vi "deeplabv3_opencv.vi"() -> ()   [LabVIEW 2018]
uses:
  <vilib>/addons/VIRobotics/opencv_yiku/ctls/ColorConversionCodes.ctl
  <vilib>/addons/VIRobotics/opencv_yiku/Mat/Mat_32F/Mat_32F.lvclass
  C:/Program Files/National Instruments/LabVIEW 2018_64bit/vi.lib/addons/VIRobotics/opencv_yiku/Mat/Mat/Mat.lvclass
  <vilib>/addons/VIRobotics/opencv_yiku/Mat/Mat_8U/Mat_8U.lvclass
  <vilib>/addons/VIRobotics/opencv_yiku/Mat/Mat/Mat_length.vi
  <vilib>/addons/VIRobotics/opencv_yiku/Mat/Mat/Mat_release.vi
  <vilib>/addons/VIRobotics/opencv_yiku/dnn/Net/Net.lvclass
  <vilib>/addons/VIRobotics/opencv_yiku/opencv_yiku.lvlib
  <vilib>/addons/VIRobotics/opencv_yiku/Mat/Mat/Mat.lvclass
panel:
  out "mask":picture
  out "原始图像":picture
  out "合成的图像":picture
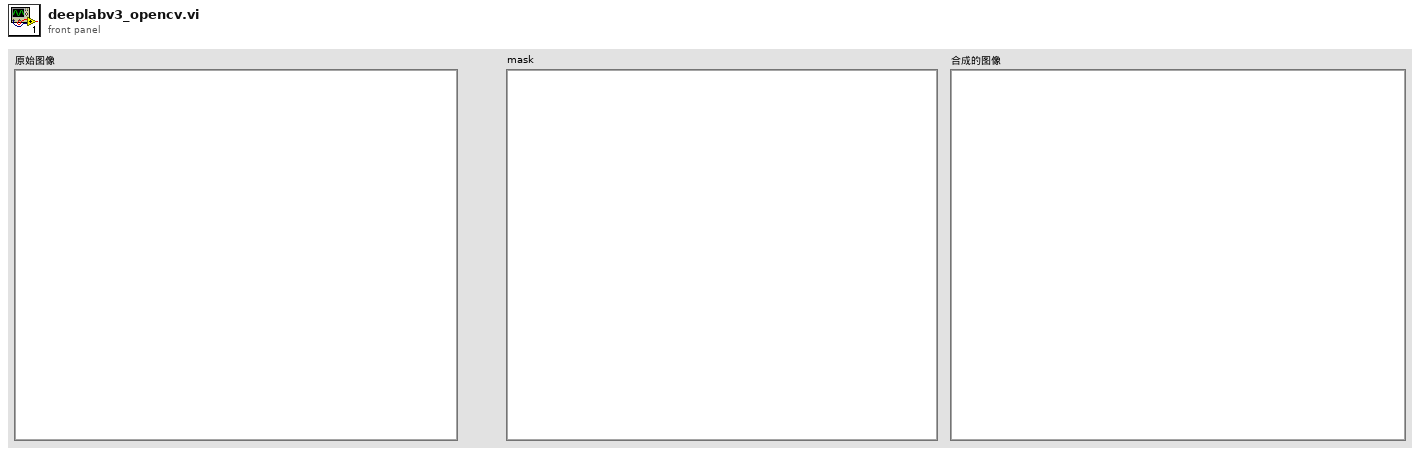
[diagram p1: front panel]
types:
  T1 = typedef "opencv_yiku.lvlib/ColorConversionCodes.ctl" = enum32{"COLOR_BGR2BGRA", "COLOR_BGRA2BGR", "COLOR_BGR2RGBA", "COLOR_RGBA2BGR", "COLOR_BGR2RGB", "COLOR_BGRA2RGBA", "COLOR_BGR2GRAY", "COLOR_RGB2GRAY", "COLOR_GRAY2BGR", "COLOR_GRAY2BGRA", "COLOR_BGRA2GRAY", "COLOR_RGBA2GRAY", "COLOR_BGR2BGR565", "COLOR_RGB2BGR565", "COLOR_BGR5652BGR", "COLOR_BGR5652RGB", "COLOR_BGRA2BGR565", "COLOR_RGBA2BGR565", "COLOR_BGR5652BGRA", "COLOR_BGR5652RGBA", "COLOR_GRAY2BGR565", "COLOR_BGR5652GRAY", "COLOR_BGR2BGR555", "COLOR_RGB2BGR555", "COLOR_BGR5552BGR", "COLOR_BGR5552RGB", "COLOR_BGRA2BGR555", "COLOR_RGBA2BGR555", "COLOR_BGR5552BGRA", "COLOR_BGR5552RGBA", "COLOR_GRAY2BGR555", "COLOR_BGR5552GRAY", "COLOR_BGR2XYZ", "COLOR_RGB2XYZ", "COLOR_XYZ2BGR", "COLOR_XYZ2RGB", "COLOR_BGR2YCrCb", "COLOR_RGB2YCrCb", "COLOR_YCrCb2BGR", "COLOR_YCrCb2RGB", "COLOR_BGR2HSV", "COLOR_RGB2HSV", "42", "43", "COLOR_BGR2Lab", "COLOR_RGB2Lab"}
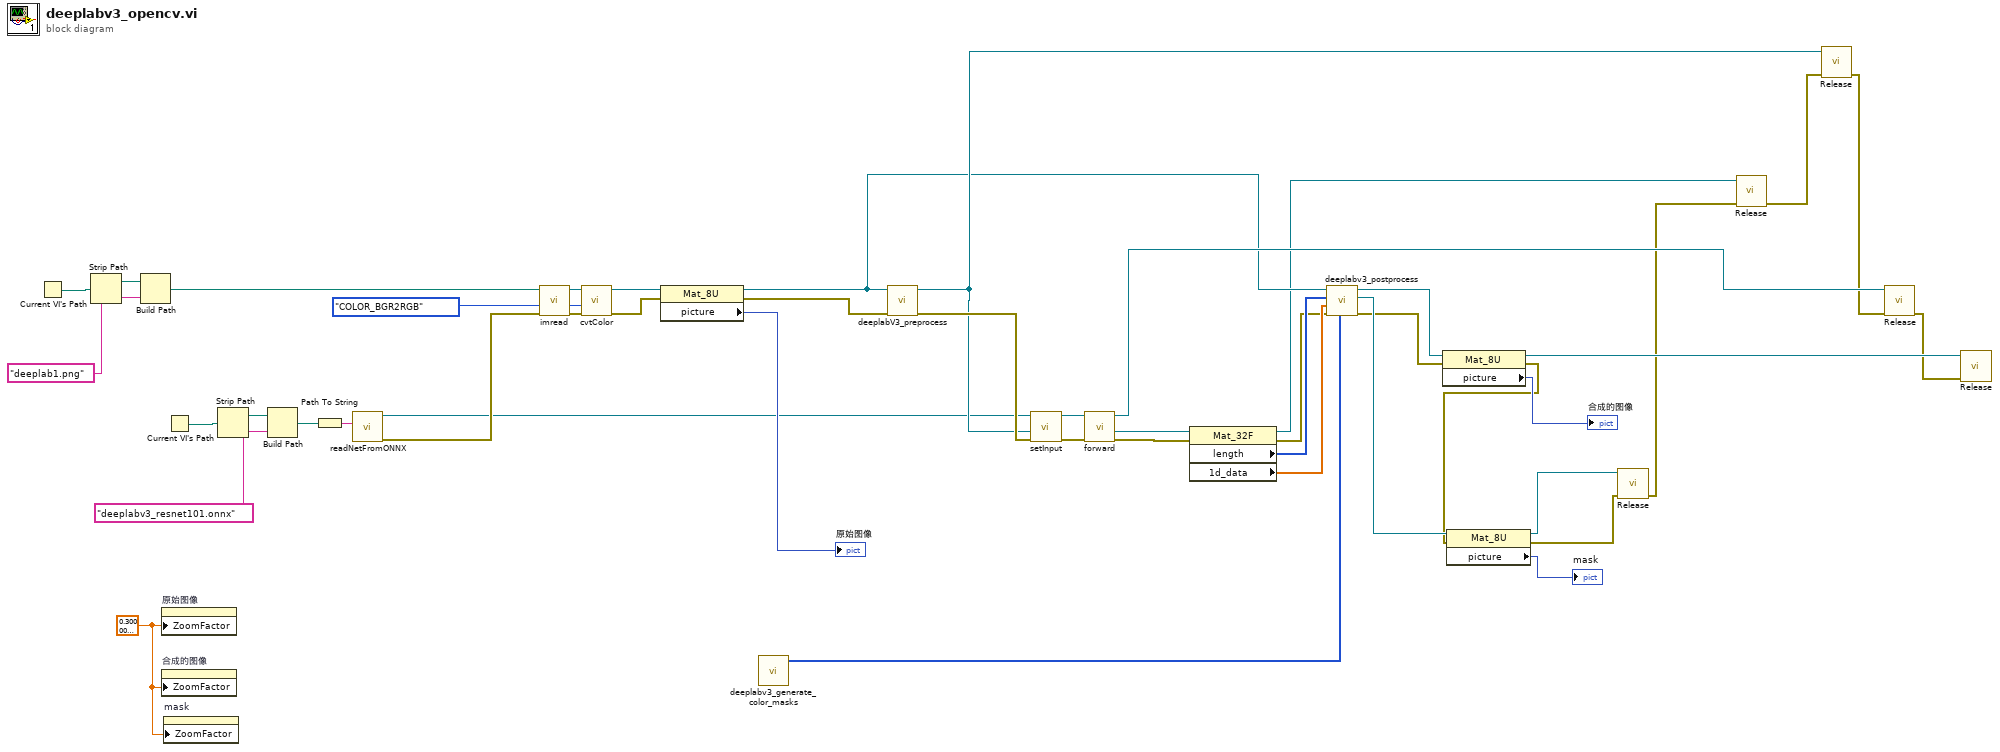
[diagram p0: block diagram]
diagram:
  w14 = sgl 0.3 ("Zoom Factor")
  n1 = Current VI's Path() -> (path=w41:path)
  n2 = Strip Path(path=w41) -> (stripped path=w42:path)  [unwired: 1 out]
  n3 = Build Path(base path=w42, name or relative path="deeplab1.png") -> (appended path=w39:path)
  n4 = property on="原始图像" class="Pict"("ZoomFactor"=w14) -> ()  [unwired: 2 in, 2 out]
  n5 = property on="合成的图像" class="Pict"("ZoomFactor"=w14) -> ()  [unwired: 2 in, 2 out]
  n6 = property on="mask" class="Pict"("ZoomFactor"=w14) -> ()  [unwired: 2 in, 2 out]
  n7 = Current VI's Path() -> (path=w37:path)
  n8 = Strip Path(path=w37) -> (stripped path=w38:path)  [unwired: 1 out]
  n9 = Build Path(base path=w38, name or relative path="deeplabv3_resnet101.onnx") -> (appended path=w35:path)
  n10 = Path To String(path=w35) -> (string=w45:string)
  n11 = call <vilib>:"readNetFromONNX.vi"("model"=w45) -> ("error out"=w43:errorcluster, "Net out"=w19:refnum<class "Net.lvclass">)  [unwired: 9 in]
  n12 = call <vilib>:"imread.vi"("error in (no error)"=w43, "path"=w39) -> ("error out"=w31:errorcluster, "Mat out"=w34:refnum<class "Mat_8U.lvclass">)  [unwired: 8 in]
  n13 = call <vilib>:"cvtColor.vi"("error in (no error)"=w31, "dstCn"=ColorConversionCodes."COLOR_BGR2RGB", "src"=w34) -> ("error out"=w23:errorcluster, "src out"=w30:refnum<class "Mat_8U.lvclass">)  [unwired: 6 in, 1 out]
  n14 = property class="Mat_8U"(reference=w30, error in=w23) -> (reference out=w22:refnum<class "Mat_8U.lvclass">, error out=w24:errorcluster, "picture"=→"原始图像":picture)
  n15 = call "deeplabv3_generate_color_masks.vi"() -> ("colors"=w1:u32[])  [unwired: 11 in]
  n16 = call "deeplabV3_preprocess.vi"("error in (no error)"=w24, "img"=w22) -> ("error out"=w32:errorcluster, "blob"=w25:refnum<class "Mat_32F.lvclass">)  [unwired: 8 in]
  n17 = call <vilib>:"setInput.vi"("error in (no error)"=w32, "Mat"=w25, "Net in"=w19) -> ("error out"=w20:errorcluster, "Net out"=w21:refnum<class "Net.lvclass">)  [unwired: 7 in]
  n18 = call <vilib>:"forward.vi"("error in (no error)"=w20, "Net in"=w21) -> ("error out"=w7:errorcluster, "Mat out"=w10:refnum<class "Mat_32F.lvclass">, "Net out"=w44:refnum<class "Net.lvclass">)  [unwired: 7 in]
  n19 = property class="Mat_32F"(reference=w10, error in=w7) -> (reference out=w5:refnum<class "Mat_32F.lvclass">, error out=w6:errorcluster, "length"=w9:i32[], "1d_data"=w8:sgl[])
  n20 = call "deeplabv3_postprocess.vi"("colors"=w1, "error in (no error)"=w6, "1d_data"=w8, "length"=w9, "img in"=w22) -> ("error out"=w12:errorcluster, "mask"=w16:refnum<class "Mat_8U.lvclass">, "img out"=w28:refnum<class "Mat_8U.lvclass">)  [unwired: 4 in]
  n21 = property class="Mat_8U"(reference=w28, error in=w12) -> (reference out=w26:refnum<class "Mat_8U.lvclass">, error out=w2:errorcluster, "picture"=→"合成的图像":picture)
  n22 = property class="Mat_8U"(reference=w16, error in=w2) -> (reference out=w13:refnum<class "Mat_8U.lvclass">, error out=w11:errorcluster, "picture"=→"mask":picture)
  n23 = call-poly <vilib>:"Release.vi"("error in (no error)"=w11, "Mat in"=w13) -> ("error out"=w3:errorcluster)  [unwired: 9 in]
  n24 = call-poly <vilib>:"Release.vi"("error in (no error)"=w3, "Mat in"=w5) -> ("error out"=w18:errorcluster)  [unwired: 9 in]
  n25 = call-poly <vilib>:"Release.vi"("error in (no error)"=w18, "Mat in"=w25) -> ("error out"=w17:errorcluster)  [unwired: 9 in]
  n26 = call-poly <vilib>:"Release.vi"("error in (no error)"=w17, "Net in"=w44) -> ("error out"=w4:errorcluster)  [unwired: 9 in]
  n27 = call-poly <vilib>:"Release.vi"("error in (no error)"=w4, "Mat in"=w26) -> ()  [unwired: 9 in, 1 out]
